vi "single_time_step.vi"(0 "Time (s)":dbl, 5 "Microwave on":bool=TRUE, 7 "Internal parameters in":T4, 9 "Fit parameters":T1, 11 "Physical constants":T3, 12 "System parameters":T2) -> (8 "Internal parameters out":T4)   [LabVIEW 2015]
uses:
  Simulation (old)/internal_parameters.ctl
  Simulation (old)/physical_constants.ctl
  Simulation (old)/system_parameters.ctl
  Simulation (old)/fit_parameters.ctl
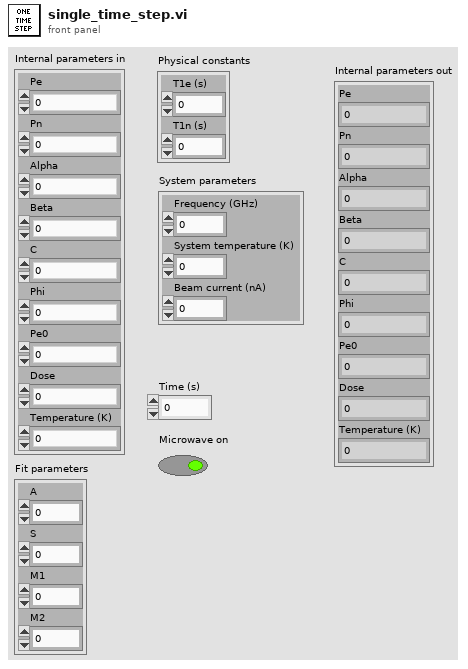
[diagram p1: front panel]
types:
  T1 = typedef "fit_parameters.ctl" = cluster{"A":dbl, "S":dbl, "M1":dbl, "M2":dbl}
  T2 = typedef "system_parameters.ctl" = cluster{"Frequency (GHz)":dbl, "System temperature (K)":dbl, "Beam current (nA)":dbl}
  T3 = typedef "physical_constants.ctl" = cluster{"T1e (s)":dbl, "T1n (s)":dbl}
  T4 = typedef "internal_parameters.ctl" = cluster{"Pe":dbl, "Pn":dbl, "Alpha":dbl, "Beta":dbl, "C":dbl, "Phi":dbl, "Pe0":dbl, "Dose":dbl, "Temperature (K)":dbl}
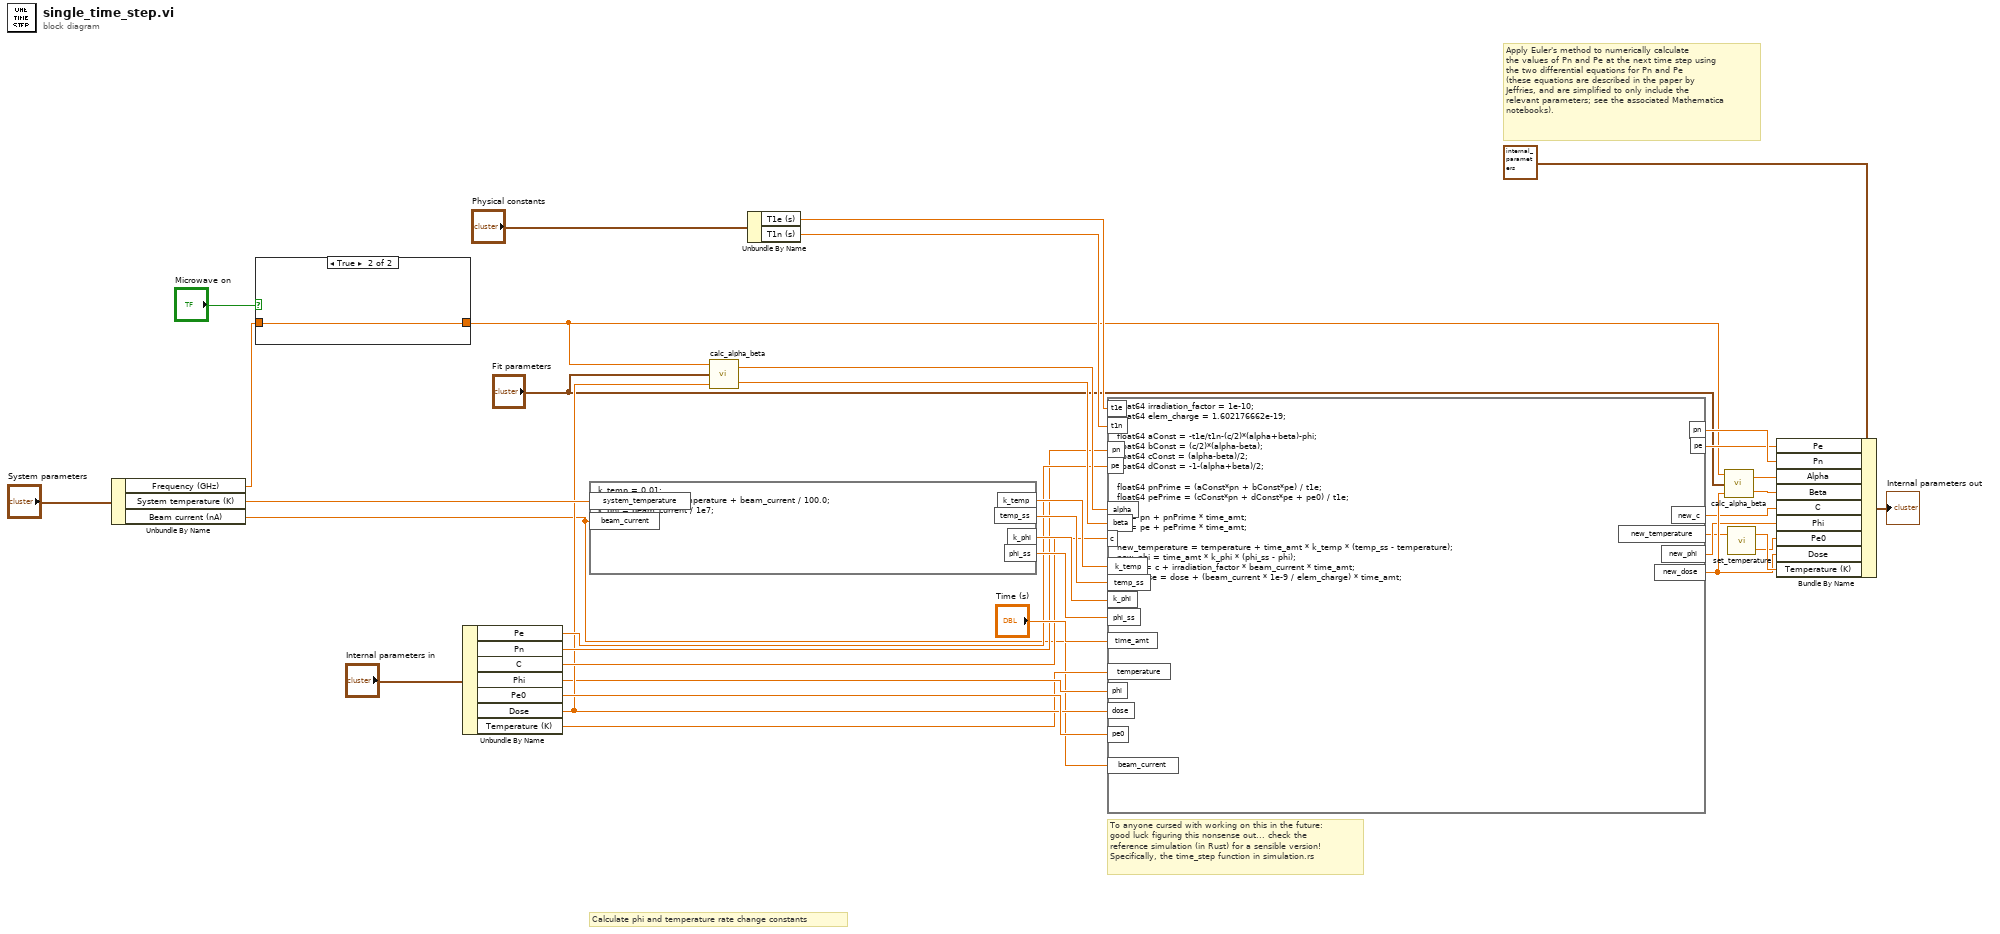
[diagram p0: block diagram]
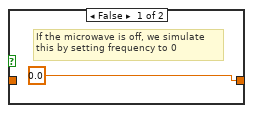
[diagram p2: hidden frame]
diagram:
  # "To anyone cursed with working on this in the future:\ngood luck figuring this nonsense out... check the\nreference simulation (in Rust) for a sensible version!\nSpecifically, the time_step function in simulation.rs"
  # "Apply Euler's method to numerically calculate\nthe values of Pn and Pe at the next time step using\nthe two differential equations for Pn and Pe\n(these equations are described in the paper by\nJeffries, and are simplified to only include the\nrelevant parameters; see the associated Mathematica\nnotebooks)."
  # "Calculate phi and temperature rate change constants"
  n1 = Unbundle By Name("System parameters") -> ("Frequency (GHz)"=w4:dbl, "System temperature (K)"=w27:dbl, "Beam current (nA)"=w17:dbl)
  n2 = case shown="True" "Microwave on" {
    tunnel: w4 -> [_ w39]
    tunnel: [0.0 ("Frequency") w39] -> w3
    frame False {
      # "If the microwave is off, we simulate\nthis by setting frequency to 0"
    }
    frame True {
    }
  }
  n3 = Unbundle By Name("Internal parameters in") -> ("Pe"=w24:dbl, "Pn"=w23:dbl, "C"=w22:dbl, "Phi"=w19:dbl, "Pe0"=w21:dbl, "Dose"=w20:dbl, "Temperature (K)"=w18:dbl)
  n4 = formula code="k_temp = 0.01;\ntemp_ss = system_temperature + beam_current / 100.0;\nk_phi = beam_current / 1e7;\nphi_ss = 0.001;"("system_temperature"=w27, "beam_current"=w17) -> ("k_temp"=w37:dbl, "temp_ss"=w36:dbl, "k_phi"=w35:dbl, "phi_ss"=w34:dbl)
  n5 = call "calc_alpha_beta.vi"("Dose"=w20, "Fit parameters"="Fit parameters", "Frequency (GHz)"=w3) -> ("Beta"=w32:dbl, "Alpha"=w33:dbl)
  n6 = Unbundle By Name("Physical constants") -> ("T1e (s)"=w26:dbl, "T1n (s)"=w25:dbl)
  n7 = formula code="float64 irradiation_factor = 1e-10;\nfloat64 elem_charge = 1.602176662e-19;\n\nfloat64 aConst = -t1e/t1n-(c/2)*(alpha+beta)-phi;\nfloat64 bConst = (c/2)*(alpha-beta);\nfloat64 cConst = (alpha-beta)/2;\nfloat64 dConst = -1-(alpha+beta)/2;\n\nfloat64 pnPrime = (aConst*pn + bConst*pe) / t1e;\nfloat64 pePrime = (cConst*pn + dConst*pe + pe0) / t1e;\n\npn = pn + pnPrime * time_amt;\npe = pe + pePrime * time_amt;\n\nnew_temperature = temperature + time_amt * k_temp * (temp_ss - temperature);\nnew_phi = time_amt * k_phi * (phi_ss - phi);\nnew_c = c + irradiation_factor * beam_current * time_amt;\nnew_dose = dose + (beam_current * 1e-9 / elem_charge) * time_amt;"("pn"=w23, "pe"=w24, "t1e"=w26, "alpha"=w33, "beta"=w32, "c"=w22, "t1n"=w25, "k_temp"=w37, "temp_ss"=w36, "k_phi"=w35, "phi_ss"=w34, "temperature"=w18, "time_amt"="Time (s)", "phi"=w19, "dose"=w20, "pe0"=w21, "beam_current"=w17) -> ("pn"=w7:dbl, "pe"=w6:dbl, "new_temperature"=w1:dbl, "new_phi"=w11:dbl, "new_dose"=w13:dbl, "new_c"=w10:dbl)
  n8 = call "calc_alpha_beta.vi"("Dose"=w13, "Fit parameters"="Fit parameters", "Frequency (GHz)"=w3) -> ("Beta"=w8:dbl, "Alpha"=w9:dbl)
  n9 = call "set_temperature.vi"("Temperature in"=w1) -> ("Pe0 out"=w12:dbl, "Temperature out"=w14:dbl)  [unwired: 1 in]
  n10 = Bundle By Name(cluster=T4 {"Pe"=0.0, "Pn"=0.0, "Alpha"=0.0, "Beta"=0.0, "C"=0.0, "Phi"=0.0, "Pe0"=0.0, "Dose"=0.0, "Temperature (K)"=0.0} ("Simulation parameters out"), "Pe"=w6, "Pn"=w7, "Alpha"=w9, "Beta"=w8, "C"=w10, "Phi"=w11, "Pe0"=w12, "Dose"=w13, "Temperature (K)"=w14) -> (→"Internal parameters out":T4)
